vi "UPRcontroller_v00_basedonlsmv66.vi"() -> ()   [LabVIEW 2015] (continued)
                          tunnel: [_ _ _ _ _ w2450 _ _ _ _] -> w2290
                          tunnel: [_ _ _ _ _ w2449 _ _ _ _] -> w2289
                          tunnel: [_ _ _ _ _ w2448 _ _ _ _] -> w2288
                          tunnel: [_ _ _ _ _ w2447 _ _ _ _] -> w2287
                          tunnel: [_ _ _ _ _ w2446 _ _ _ _] -> w2286
                          tunnel: [_ _ _ _ _ w2445 _ _ _ _] -> w2285
                          tunnel: [_ _ _ _ _ w2444 _ _ _ _] -> w2284
                          tunnel: [_ _ _ _ _ w2443 _ _ _ _] -> w2283
                          frame #0 {
                            n108 = local read "Auto Shutter Channels"() -> (w2304:i32[])
                            n109 = local read "AI channels"() -> (w2310:i32[])
                            n110 = local read "CI channels"() -> (w2309:i32[])
                            n111 = call "2pparameters.vi"("command"="get") -> ("params out"=w2307:T12)  [unwired: 1 in]
                            n112 = Bundle By Name(cluster=w2307, "aAI"=w2310, "aCI"=w2309, "aAS"=w2304) -> (w2308:T12)
                            n113 = call "2pparameters.vi"("Params in"=w2308, "command"="set") -> ()  [unwired: 1 out]
                          }
                          frame #1 {
                            n114 = local read "Vy-min ref"() -> (w2315:dbl)
                            n115 = local read "Vy-max ref"() -> (w2316:dbl)
                            n116 = local read "Angle ref"() -> (w2314:dbl)
                            n117 = local read "Vx-min ref"() -> (w2317:dbl)
                            n118 = local write "counts"(0 ("counts")) -> ()
                            n119 = local write "graphtab"(T5."image" ("graphtab")) -> ()
                            n120 = local read "Vx-max ref"() -> (w2318:dbl)
                            n121 = property on="Stop" class="Bool (strict)"("Visible"=TRUE, "DisabledEnum"=T8."Enabled" ("Disabled")) -> ()  [unwired: 2 in, 2 out]
                            n122 = property on="Start" class="Bool (strict)"("Visible"=FALSE, "DisabledEnum"=T8."Disabled and Grayed Out" ("Disabled")) -> ()  [unwired: 2 in, 2 out]
                            n123 = script code="Xic=(ximax+ximin)./2;\nYic=(yimax+yimin)./2;\nximin=ximin-Xic;\nymin=ymin-Yic;\nxirmin=ximin.*cos(pi/180.*phi)+yimin.*sin(pi./180.*phi)+Xic;\nyirmin=-ximin.*sin(pi./180.*phi)+yimin.*cos(pi./180.*phi)+Yic;"("ximax"=w2318, "ximin"=w2317, "yimax"=w2316, "yimin"=w2315, "phi"=w2314) -> ("xirmin"=w2313:dbl, "yirmin"=w2312:dbl)  [unwired: 1 in, 1 out]
                            n124 = stacked-sequence {
                              tunnel: w2311 -> [_ w2343 _]
                              frame #0 {
                                n125 = local read "Measurement"() -> (w2325:T4)
                                n126 = case shown="\"X-Y-t movie\", Default" w2325 {
                                frame "X-Y-t movie", Default {
                                n127 = call "2pparameters.vi"("command"="get") -> ("params out"=w2328:T12)  [unwired: 1 in]
                                n128 = Bundle By Name(cluster=w2328, "type"="X-Y-t movie") -> (w2326:T12)
                                n129 = call "2pparameters.vi"("Params in"=w2326, "command"="set") -> ()  [unwired: 1 out]
                                }
                                frame "X-Y-Z stack" {
                                n130 = call "2pparameters.vi"("command"="get") -> ("params out"=w2333:T12)  [unwired: 1 in]
                                n131 = Bundle By Name(cluster=w2333, "type"="X-Y-Z stack") -> (w2331:T12)
                                n132 = call "2pparameters.vi"("Params in"=w2331, "command"="set") -> ()  [unwired: 1 out]
                                }
                                frame "Lifetime (scan)" {
                                n133 = call "2pparameters.vi"("command"="get") -> ("params out"=w2338:T12)  [unwired: 1 in]
                                n134 = Bundle By Name(cluster=w2338, "type"="Lifetime (scan)") -> (w2336:T12)
                                n135 = call "2pparameters.vi"("Params in"=w2336, "command"="set") -> ()  [unwired: 1 out]
                                }
                                }
                              }
                              frame #1 {
                                n136 = Format Date/Time String(time format string (%c)="%Y%m%d", seconds (now)=w2343) -> (date/time string=w2342:string)  [unwired: 1 in]
                                n137 = Format Date/Time String(time format string (%c)="%H%M%S", seconds (now)=w2343) -> (date/time string=w2341:string)  [unwired: 1 in]
                                n138 = call "2pparameters.vi"("command"="get") -> ("params out"=w2347:T12)  [unwired: 1 in]
                                n139 = Bundle By Name(cluster=w2347, "date"=w2342, "time"=w2341) -> (w2346:T12)
                                n140 = call "2pparameters.vi"("Params in"=w2346, "command"="set") -> ()  [unwired: 1 out]
                              }
                              frame #2 {
                                n141 = call "configuration.vi"("command"="get") -> ("config out"=w2357:T14)  [unwired: 2 in, 1 out]
                                n142 = Unbundle By Name(w2357) -> ("CI names"=w2358:string[], "AI names"=w2359:string[])
                                n143 = call "2pparameters.vi"("command"="get") -> ("params out"=w2353:T12)  [unwired: 1 in]
                                n144 = Unbundle By Name(w2353) -> ("aCI"=w2354:i32[], "aAI"=w2355:i32[])
                                n145 = for {
                                tunnel: w2354 -> [w2369] mode=indexing
                                tunnel: w2358 -> [w2370]
                                tunnel: [w2368] -> w2360 mode=indexing
                                n146 = Index Array(array=w2370, index=w2369) -> (element=w2368:string)
                                }
                                n147 = for {
                                tunnel: w2355 -> [w2366] mode=indexing
                                tunnel: w2359 -> [w2367]
                                tunnel: [w2365] -> w2361 mode=indexing
                                n148 = Index Array(array=w2367, index=w2366) -> (element=w2365:string)
                                }
                                n149 = Build Array (concatenate)(w2360, w2361) -> (w2351:string[])
                                n150 = for {
                                tunnel: w2351 -> [w2363] mode=indexing
                                tunnel: [w2362] -> w2350 mode=indexing
                                i -> [w2364]
                                n151 = Bundle("String"=w2363, w2364) -> (w2362:cluster{"String":string, i32})  [unwired: 1 in]
                                }
                                n152 = property on="image2list" class="Ring (strict)"("StringsAndValues[]"=w2350) -> ()  [unwired: 2 in, 2 out]
                                n153 = property on="image1list" class="Ring (strict)"("StringsAndValues[]"=w2350) -> ()  [unwired: 2 in, 2 out]
                                n154 = property on="image1list chB" class="Ring (strict)"("StringsAndValues[]"=w2350) -> ()  [unwired: 2 in, 2 out]
                                n155 = property on="image1list chA" class="Ring (strict)"("StringsAndValues[]"=w2350) -> ()  [unwired: 2 in, 2 out]
                              }
                            }
                            n156 = call "setposition.vi"("Vy"=w2312, "Vx"=w2313) -> ()  [unwired: 1 in]
                          }
                          frame #2 {
                            n157 = call "X-array-databuffer.vi"("command"=enum16{"get", "set", "clear", "append"}."clear") -> ()  [unwired: 3 in, 2 out]
                            n158 = call "Y-array-databuffer.vi"("command"=enum16{"get", "set", "clear", "append"}."clear") -> ()  [unwired: 3 in, 2 out]
                            n159 = call "2pparameters.vi"("command"="get") -> ("params out"=w2374:T12)  [unwired: 1 in]
                            n160 = Unbundle By Name(w2374) -> ("aAS"=w2371:u32[], "autoshutter"=w2375:bool, "auto OD"=w2372:bool)
                            n161 = call "allAI-temp_img.vi"("command"=enum16{"get", "set", "clear", "append"}."clear") -> ()  [unwired: 3 in, 2 out]
                            n162 = case shown="True" w2372 {
                              frame False {
                              }
                              frame True {
                                n163 = call "configuration.vi"("command"="get") -> ("config out"=w2383:T14)  [unwired: 2 in, 1 out]
                                n164 = Unbundle By Name(w2383) -> ("image OD"=w2384:u16)
                                n165 = local read "ODfilt"() -> (w2381:u16)
                                n166 = call "filterwheelcontrol_nothorlabslib.vi"("Current OD filt"=w2381, "New ODfilt"=w2384) -> ()  [unwired: 1 in]
                              }
                            }
                            n167 = case shown="True" w2375 {
                              tunnel: w2371 -> [_ w2385]
                              frame False {
                              }
                              frame True {
                                n168 = call "shuttercontrol_multi.vi"("Autoshutter Chans"=w2385, "command"="close") -> ()  [unwired: 1 in, 1 out]
                              }
                            }
                            n169 = call "CH1-temp.vi"("command"=enum16{"get", "set", "clear", "add row"}."clear") -> ()  [unwired: 3 in, 2 out]
                            n170 = call "CH2-temp.vi"("command"=enum16{"get", "set", "clear", "add row"}."clear") -> ()  [unwired: 3 in, 2 out]
                          }
                          frame #3 {
                            n171 = local read "avpp"() -> (w2419:i32)
                            n172 = local read "Angle ref"() -> (w2418:dbl)
                            n173 = local read "ROI Type"() -> (w2417:u16)
                            n174 = local read "xpixels ref"() -> (w2414:i32)
                            n175 = local read "Vx-min ref"() -> (w2413:dbl)
                            n176 = local read "Vx-max ref"() -> (w2412:dbl)
                            n177 = local read "ypixels ref"() -> (w2410:i32)
                            n178 = local read "Vy-min ref"() -> (w2411:dbl)
                            n179 = local read "Vy-max ref"() -> (w2407:dbl)
                            n180 = local read "Sampling rate"() -> (w2401:dbl)
                            n181 = local read "finite samples"() -> (w2402:bool)
                            n182 = local read "continuous"() -> (w2405:bool)
                            n183 = local read "wavdet"() -> (w2406:bool)
                            n184 = local read "# of frames"() -> (w2404:i32)
                            n185 = local read "maxbufferAI"() -> (w2403:i32)
                            n186 = local read "Override AI buffer"() -> (w2387:bool)
                            n187 = call "2pparameters.vi"("command"="get") -> ("params out"=w2416:T12)  [unwired: 1 in]
                            n188 = Bundle By Name(cluster=w2416, "avpp"=w2419, "Angle Img"=w2418, "Xpixels Img"=w2414, "Vx-min Img"=w2413, "VX-max Img"=w2412, "Ypixels Img"=w2410, "Vy-min Img"=w2411, "Vy-max Img"=w2407, "srate"=w2401, "srate Img"=w2401, "finite"=w2402, "cont"=w2405, "wavdet"=w2406, "measpoints"=w2404, "maxbufferAI"=w2403, "Drawing Mode"=w2417, "Vz-reset"=0.0, "AIoverride"=w2387) -> (w2408:T12)
                            n189 = call "2pparameters.vi"("Params in"=w2408, "command"="set") -> ()  [unwired: 1 out]
                            n190 = local read "Vholding (mV)"() -> (w2390:sgl)
                            n191 = local read "OCgain"() -> (w2391:sgl)
                            n192 = local read "holdon"() -> (w2389:bool)
                            n193 = local read "Current Clamp"() -> (w2396:bool)
                            n194 = local read "Voltage Clamp"() -> (w2395:bool)
                            n195 = local read "CC_ICgain"() -> (w2394:dbl)
                            n196 = call "patchparameters.vi"("command"="get") -> ("Params out"=w2398:T16)  [unwired: 1 in]
                            n197 = Bundle By Name(cluster=w2398, "VC"=w2395, "CC"=w2396, "CC_icg (pA/mv)"=w2394, "VC_icg (mV/mV)"=sgl 10.0, "OCG (mV/pA)"=w2391, "OVG (mV/mV)"=0.1, "Vhold (mV)"=w2390, "holdon"=w2389) -> (w2397:T16)
                            n198 = call "patchparameters.vi"("Params in"=w2397, "command"="set") -> ()  [unwired: 1 out]
                          }
                          frame #4 {
                            # "these store the actual scanning waveforms (for one iteration)"
                            # "Generate Waveforms for Scanning Mirrors"
                            # "Creates The scanning waveform here"
                            n199 = call "2pparameters.vi"("command"="get") -> ("params out"=w2434:T12)  [unwired: 1 in]
                            n200 = Unbundle By Name(w2434) -> ("srate Img"=w2433:sgl, "Angle Img"=w2432:dbl, "VX-max Img"=w2431:dbl, "Vx-min Img"=w2430:dbl, "Xpixels Img"=w2429:i32, "Ypixels Img"=w2428:i32, "Vy-max Img"=w2427:dbl, "Vy-min Img"=w2426:dbl, "Drawing Mode"=w2425:u16)
                            n201 = call "ROI-databuffer.vi"("command"=enum16{"get", "set", "clear", "append"}."get") -> ("array out"=w2424:cluster{"x":sgl, "y":sgl}[])  [unwired: 4 in]
                            n202 = call "ScanningWaveform_v4.vi"("Vy-min"=w2426, "Vy-max"=w2427, "yPixels/tPixels"=w2428, "xPixels/rPixels"=w2429, "Vx-min"=w2430, "Vx-max"=w2431, "Drawing Mode"=w2425, "Angle"=w2432, "AOrate"=w2433, "Points"=w2424) -> ("numPixels"=w2420:dbl, "Y-WaveArray"=w2423:dbl[], "P"=w2421:dbl, "X-WaveArray"=w2422:dbl[])  [unwired: 6 in]
                            n203 = call "2pparameters.vi"("command"="get") -> ("params out"=w2442:T12)  [unwired: 1 in]
                            n204 = call "Y-array-databuffer.vi"("array in"=w2423, "command"=enum16{"get", "set", "clear", "append"}."set") -> ()  [unwired: 2 in, 2 out]
                            n205 = call "X-array-databuffer.vi"("array in"=w2422, "command"=enum16{"get", "set", "clear", "append"}."set") -> ()  [unwired: 2 in, 2 out]
                            n206 = Bundle By Name(cluster=w2442, "P"=w2421, "sAOxy"=w2420) -> (w2439:T12)
                            n207 = call "2pparameters.vi"("Params in"=w2439, "command"="set") -> ()  [unwired: 1 out]
                          }
                          frame #5 {
                            # "rem2Ps"
                            # "A2Ps"
                            # "Al"
                            # "Rl"
                            # "Combines scanning waveform with \"wavform generation\" waveforms"
                            n208 = stacked-sequence {
                              seq-local: [w2461 _ _ _ _ _ _ _ _ _ _] -> [_ w2581 _ w2636 _ w2716 _ _ _ _ _]
                              seq-local: [w2462 _ _ _ _ _ _ _ _ _ _] -> [_ w2582 w2592 _ w2685 _ _ _ _ _ _]
                              seq-local: [_ _ w2591 _ _ _ _ _ _ _ _] -> [_ _ _ _ w2679 _ _ _ _ _ _]
                              seq-local: [_ _ _ w2635 _ _ _ _ _ _ _] -> [_ _ _ _ _ w2715 _ _ _ _ _]
                              seq-local: [w2458 _ _ _ _ _ _ _ _ _ _] -> [_ w2578 _ _ _ _ _ _ w2925 w2993 _]
                              seq-local: [w2457 _ _ _ _ _ _ _ _ _ _] -> [_ w2577 _ _ _ _ _ _ w2926 w2994 _]
                              seq-local: [w2464 _ _ _ _ _ _ _ _ _ _] -> [_ _ _ _ _ _ w2754 _ w2924 w2992 _]
                              seq-local: [w2460 _ _ _ _ _ _ _ _ _ _] -> [_ w2576 _ _ _ _ w2753 w2832 _ _ _]
                              seq-local: [w2459 _ _ _ _ _ _ _ _ _ _] -> [_ w2575 _ _ _ _ w2752 w2831 _ _ _]
                              seq-local: [w2463 _ _ _ _ _ _ _ _ _ _] -> [_ _ _ _ _ _ w2751 w2830 _ _ _]
                              tunnel: [_ _ w2590 _ _ _ _ _ _ _ _] -> w2455
                              tunnel: [_ _ w2589 _ _ _ _ _ _ _ _] -> w2454
                              tunnel: [w2462 _ _ _ _ _ _ _ _ _ _] -> w2456
                              tunnel: [w2461 _ _ _ _ _ _ _ _ _ _] -> w2453
                              tunnel: [_ _ _ w2634 _ _ _ _ _ _ _] -> w2452
                              tunnel: [_ _ _ w2633 _ _ _ _ _ _ _] -> w2451
                              tunnel: [w2460 _ _ _ _ _ _ _ _ _ _] -> w2450
                              tunnel: [w2459 _ _ _ _ _ _ _ _ _ _] -> w2449
                              tunnel: [_ _ _ _ _ _ w2750 _ _ _ _] -> w2448
                              tunnel: [_ _ _ _ _ _ _ w2829 _ _ _] -> w2447
                              tunnel: [w2458 _ _ _ _ _ _ _ _ _ _] -> w2446
                              tunnel: [w2457 _ _ _ _ _ _ _ _ _ _] -> w2445
                              tunnel: [_ _ _ _ _ _ _ _ w2923 _ _] -> w2444
                              tunnel: [_ _ _ _ _ _ _ _ _ w2991 _] -> w2443
                              frame #0 {
                                # "channels\nadded/removed"
                                # "all these arrows go to frames\n6 and 7"
                                # "for a next version, give ome thought to\nthe possibilit of intermittently updating the\nwaveforms. it will have to be a calculation\nbased on speed of CPU and program on the one hand\nand length of measurement on the other. but then it should be possible, in principle, to \nupdate the waveform on the fly and that way cut up a longer measurement in smaller parts."
                                # "Y"
                                # "X"
                                # "This frame takes channels from \"waveform generation\" and adds, X,Y,2p shutter and Lifetime Timestamp (if those where not manually defined in WG)"
                                n209 = stacked-sequence {
                                tunnel: [w2465 _ _ _] -> w2462
                                tunnel: [_ w2477 _ _] -> w2461
                                tunnel: [_ _ _ w2542] -> w2457
                                tunnel: [_ _ _ w2541] -> w2458
                                tunnel: [_ _ _ w2540] -> w2464
                                tunnel: [_ _ w2492 _] -> w2460
                                tunnel: [_ _ w2491 _] -> w2459
                                tunnel: [_ _ w2490 _] -> w2463
                                frame #0 {
                                n210 = call "configuration.vi"("command"="get") -> ("config out"=w2467:T14)  [unwired: 2 in, 1 out]
                                n211 = Unbundle By Name(w2467) -> ("Voltage to Xgalvo"=w2466:i32)
                                n212 = call "2pparameters.vi"("command"="get") -> ("params out"=w2471:T12)  [unwired: 1 in]
                                n213 = in-place {
                                in-place-border: w2466 -> [w2476]
                                in-place-border: [w2473] -> w2465
                                n214 = in-place-cluster #1(w2471) -> ("aAO"=w2475:u32[])
                                n215 = call "add channel to active arrayv2.vi"("line array in"=w2475, "line to add"=w2476) -> ("line array out"=w2474:u32[], "addition"=w2473:bool)  [unwired: 1 out]
                                n216 = in-place-cluster #1("aAO"=w2474) -> (w2469:T12)
                                }
                                n217 = call "2pparameters.vi"("Params in"=w2469, "command"="set") -> ()  [unwired: 1 out]
                                }
                                frame #1 {
                                n218 = call "configuration.vi"("command"="get") -> ("config out"=w2479:T14)  [unwired: 2 in, 1 out]
                                n219 = Unbundle By Name(w2479) -> ("Voltage to Ygalvo"=w2478:i32)
                                n220 = call "2pparameters.vi"("command"="get") -> ("params out"=w2483:T12)  [unwired: 1 in]
                                n221 = in-place {
                                in-place-border: w2478 -> [w2488]
                                in-place-border: [w2485] -> w2477
                                n222 = in-place-cluster #2(w2483) -> ("aAO"=w2487:u32[])
                                n223 = call "add channel to active arrayv2.vi"("line array in"=w2487, "line to add"=w2488) -> ("line array out"=w2486:u32[], "addition"=w2485:bool)  [unwired: 1 out]
                                n224 = in-place-cluster #2("aAO"=w2486) -> (w2481:T12)
                                }
                                n225 = call "2pparameters.vi"("Params in"=w2481, "command"="set") -> ()  [unwired: 1 out]
                                }
                                frame #2 {
                                n226 = call "2pparameters.vi"("command"="get") -> ("params out"=w2494:T12)  [unwired: 1 in]
                                n227 = Unbundle By Name(w2494) -> ("autoshutter"=w2493:bool, "wavdet"=w2489:bool)
                                n228 = case shown="False" w2493 {
                                tunnel: [w2499 w2522] -> w2492
                                tunnel: [w2498 FALSE ("removal")] -> w2491
                                tunnel: [w2497 w2521] -> w2490
                                tunnel: w2489 -> [w2496 _]
                                frame False {
                                n229 = case shown="False" w2496 {
                                tunnel: [FALSE ("addition") FALSE ("addition")] -> w2499
                                tunnel: [w2503 FALSE ("removal")] -> w2498
                                tunnel: [w2502 _] -> w2497
                                frame False {
                                n230 = call "2pparameters.vi"("command"="get") -> ("params out"=w2501:T12)  [unwired: 1 in]
                                n231 = Unbundle By Name(w2501) -> ("aAS"=w2500:u32[])
                                n232 = in-place {
                                in-place-border: [w2508] -> w2503
                                in-place-border: [w2511] -> w2502
                                in-place-border: w2500 -> [w2510]
                                n233 = in-place-cluster #3(w2501) -> ("aDO"=w2513:u32[])
                                n234 = for {
                                tunnel: [w2516] -> w2509 mode=indexing
                                tunnel: [w2515] -> w2511 mode=indexing
                                shift-right: [w2517] -> w2512
                                shift-left: w2513 -> [w2518]
                                tunnel: w2510 -> [w2514] mode=indexing
                                n235 = call "remove channel from active arrayv2.vi"("line array in"=w2518, "line to remove"=w2514) -> ("line array out"=w2517:u32[], "removal"=w2516:bool, "index"=w2515:i32)
                                }
                                n236 = Or Array Elements(Boolean array=w2509) -> (logical OR=w2508:bool)
                                n237 = in-place-cluster #3("aDO"=w2512) -> (w2504:T12)
                                }
                                n238 = call "2pparameters.vi"("Params in"=w2504, "command"="set") -> ()  [unwired: 1 out]
                                }
                                frame True {
                                }
                                }
                                }
                                frame True {
                                n239 = call "2pparameters.vi"("command"="get") -> ("params out"=w2524:T12)  [unwired: 1 in]
                                n240 = Unbundle By Name(w2524) -> ("aAS"=w2523:u32[])
                                n241 = in-place {
                                in-place-border: w2523 -> [w2534]
                                in-place-border: [w2530] -> w2522
                                in-place-border: [w2529] -> w2521
                                n242 = in-place-cluster #4(w2524) -> ("aDO"=w2533:u32[])
                                n243 = for {
                                tunnel: w2534 -> [w2539] mode=indexing
                                shift-right: [w2537] -> w2532
                                shift-left: w2533 -> [w2538]
                                tunnel: [w2536] -> w2531 mode=indexing
                                tunnel: [w2535] -> w2529 mode=indexing
                                n244 = call "add channel to active arrayv2.vi"("line array in"=w2538, "line to add"=w2539) -> ("line array out"=w2537:u32[], "addition"=w2536:bool, "index"=w2535:i32)
                                }
                                n245 = Or Array Elements(Boolean array=w2531) -> (logical OR=w2530:bool)
                                n246 = in-place-cluster #4("aDO"=w2532) -> (w2526:T12)
                                }
                                n247 = call "2pparameters.vi"("Params in"=w2526, "command"="set") -> ()  [unwired: 1 out]
                                }
                                }
                                }
                                frame #3 {
                                n248 = local read "Measurement"() -> (w2543:T4)
                                n249 = To Unsigned Long Integer(number=w2543) -> (unsigned 32bit integer=w2544:u32)
                                n250 = case shown="5..7" w2544 {
                                tunnel: [FALSE ("addition") w2562] -> w2542
                                tunnel: [w2547 FALSE ("removal")] -> w2541
                                tunnel: [w2545 w2560] -> w2540
                                frame 0..4, Default {
                                n251 = call "configuration.vi"("command"="get") -> ("config out"=w2553:T14)  [unwired: 2 in, 1 out]
                                n252 = Unbundle By Name(w2553) -> ("LT timestamp"=w2550:u32)
                                n253 = call "2pparameters.vi"("command"="get") -> ("params out"=w2551:T12)  [unwired: 1 in]
                                n254 = in-place {
                                in-place-border: w2550 -> [w2559]
                                in-place-border: [w2556] -> w2547
                                in-place-border: [w2555] -> w2545
                                n255 = in-place-cluster #5(w2551) -> ("aDO"=w2558:u32[])
                                n256 = call "remove channel from active arrayv2.vi"("line array in"=w2558, "line to remove"=w2559) -> ("line array out"=w2557:u32[], "removal"=w2556:bool, "index"=w2555:i32)
                                n257 = in-place-cluster #5("aDO"=w2557) -> (w2548:T12)
                                }
                                n258 = call "2pparameters.vi"("Params in"=w2548, "command"="set") -> ()  [unwired: 1 out]
                                }
                                frame 5..7 {
                                n259 = call "configuration.vi"("command"="get") -> ("config out"=w2568:T14)  [unwired: 2 in, 1 out]
                                n260 = Unbundle By Name(w2568) -> ("LT timestamp"=w2565:u32)
                                n261 = call "2pparameters.vi"("command"="get") -> ("params out"=w2566:T12)  [unwired: 1 in]
                                n262 = in-place {
                                in-place-border: w2565 -> [w2574]
                                in-place-border: [w2571] -> w2562
                                in-place-border: [w2570] -> w2560
                                n263 = in-place-cluster #6(w2566) -> ("aDO"=w2573:u32[])
                                n264 = call "add channel to active arrayv2.vi"("line array in"=w2573, "line to add"=w2574) -> ("line array out"=w2572:u32[], "addition"=w2571:bool, "index"=w2570:i32)
                                n265 = in-place-cluster #6("aDO"=w2572) -> (w2563:T12)
                                }
                                n266 = call "2pparameters.vi"("Params in"=w2563, "command"="set") -> ()  [unwired: 1 out]
                                }
                                }
                                }
                                }
                              }
                              frame #1 {
                                # "Prepares the actual AO and DO lines that are going to be used for the task"
                                n267 = Or(x=w2581, y=w2582) -> (x .or. y?=w2580:bool)
                                n268 = case shown="True" w2580 {
                                frame False {
                                }
                                frame True {
                                # "update GUI"
                                n269 = call "Used AO lines.vi"() -> ("used AO names"=w2586:string[], "used AO lines"=w2588:tag[])  [unwired: 2 in]
                                n270 = control-ref of="Analog Lines Plot"() -> (w2587:refnum<vi>)
                                n271 = local write "Analog Used Lines"(w2588) -> ()
                                n272 = local write "Analog Used Names"(w2586) -> ()
                                n273 = call "prepAOWaveplot.vi"("WaveformGraph in"=w2587, "Analog Used Names"=w2586) -> ()  [unwired: 1 in]
                                }
                                }
                                n274 = Compound Arithmetic op=OR(w2578, w2577, w2576, w2575) -> (w2579:bool)
                                n275 = case shown="True" w2579 {
                                frame False {
                                }
                                frame True {
                                n276 = control-ref of="Digital Lines Plot"() -> (w2583:refnum<vi>)
                                n277 = call "Used DO lines.vi"() -> ("used DO names"=w2584:string[], "used DO lines"=w2585:tag[])  [unwired: 2 in]
                                n278 = local write "Digital Used Lines"(w2585) -> ()
                                n279 = local write "Digital Used Names"(w2584) -> ()
                                n280 = call "prepDOWaveplot.vi"("DigitalGraph in"=w2583, "used DO names"=w2584) -> ()  [unwired: 1 in]
                                }
                                }
                              }
                              frame #2 {
                                # "Make sure that the parameters used to create waveform are saved in the right format"
                                n281 = case shown="False" w2592 {
                                tunnel: [w2595 w2616] -> w2591
                                tunnel: [w2594 w2614] -> w2590
                                tunnel: [w2593 _] -> w2589
                                frame False {
                                n282 = stacked-sequence {
                                seq-local: [w2597 _] -> [_ w2610]
                                tunnel: [w2597 _] -> w2595
                                tunnel: [w2600 _] -> w2594
                                tunnel: [w2596 _] -> w2593
                                frame #0 {
                                n283 = call "configuration.vi"("command"="get") -> ("config out"=w2608:T14)  [unwired: 2 in, 1 out]
                                n284 = call "waveformparamsv2.vi"("command"="get") -> ("Params out"=w2602:T17)  [unwired: 4 in, 2 out]
                                n285 = Unbundle By Name(w2608) -> ("Voltage to Xgalvo"=w2609:i32)
                                n286 = call "2pparameters.vi"("command"="get") -> ("params out"=w2605:T12)  [unwired: 1 in]
                                n287 = Unbundle By Name(w2602) -> ("AO parameters"=w2601:T18)
                                n288 = Unbundle By Name(w2605) -> ("aAO"=w2606:u32[])
                                n289 = call "waveformsAObuffer.vi"("command"="get") -> ("AO wf out"=w2598:waveform(dbl)[])  [unwired: 1 in]
                                n290 = Search 1D Array(1D array=w2606, element=w2609) -> (index of element=w2597:i32)  [unwired: 1 in]
                                n291 = Index Array(array=w2598, index=w2597) -> (element=w2596:waveform(dbl))
                                n292 = Index Array(array=w2601, index=w2597) -> (element=w2600:T19)
                                }
                                frame #1 {
                                w2611 = 0.0 ("Step size (V)")
                                n293 = local read "Sampling rate"() -> (w2612:dbl)
                                n294 = call "replace AO XYwfparam.vi"("Baseline (V)"=w2611, "Start amplitude (V)"=w2611, "Cycles"=w2611, "Repeats"=w2611, "index of AO wave"=w2610, "Step size (V)"=w2611, "DC (%)"=w2611, "Sampling frequency (Hz)"=w2612, "Period (ms)"=w2611, "Cycle length (s)"=w2611, "Pulses"=w2611, "padding value"=w2611, "Matlab wave name"=path "xwave") -> ()  [unwired: 3 in]
                                }
                                }
                                }
                                frame True {
                                w2615 = 0.0 ("Repeats")
                                n295 = local read "Sampling rate"() -> (w2624:dbl)
                                n296 = call "2pparameters.vi"("command"="get") -> ("params out"=w2618:T12)  [unwired: 1 in]
                                n297 = call "configuration.vi"("command"="get") -> ("config out"=w2621:T14)  [unwired: 2 in, 1 out]
                                n298 = call "waveformparamsv2.vi"("command"="get") -> ("Params out"=w2630:T17)  [unwired: 4 in, 2 out]
                                n299 = Unbundle By Name(w2621) -> ("Voltage to Xgalvo"=w2622:i32)
                                n300 = Unbundle By Name(w2630) -> ("AO parameters"=w2627:T18)
                                n301 = Unbundle By Name(w2618) -> ("aAO"=w2619:u32[])
                                n302 = Search 1D Array(1D array=w2619, element=w2622) -> (index of element=w2616:i32)  [unwired: 1 in]
                                n303 = Index Array(array=w2627, index=0) -> (element=w2628:T19)
                                n304 = Bundle By Name(cluster=w2628, "AOtab"=-1.0 ("Repeats"), "Repeats"=w2615, "Cycles"=w2615, "Start amplitude (V)"=w2615, "Baseline (V)"=w2615, "Step size (V)"=w2615, "DC (%)"=w2615, "Sampling frequency (Hz)"=w2624, "Period (ms)"=w2615, "Offset (V)"=w2615, "Amplitude (V)"=w2615, "Frequency"=w2615, "Tri Repeats"=w2615, "phase shift (ms)"=w2615, "Pulses"=w2615, "Matlab wave file"=path "xwave", "padding value"=w2615) -> (w2614:T19)
                                n305 = Build Array(w2614) -> (w2625:T18)
                                n306 = call "waveformparamsv2.vi"("command"="add AO", "add AO"=w2625) -> ()  [unwired: 3 in, 3 out]
                                }
                                }
                              }
                              frame #3 {
                                n307 = case shown="False" w2636 {
                                tunnel: [w2639 w2660] -> w2635
                                tunnel: [w2638 w2658] -> w2634
                                tunnel: [w2637 _] -> w2633
                                frame False {
                                n308 = stacked-sequence {
                                seq-local: [w2641 _] -> [_ w2654]
                                tunnel: [w2641 _] -> w2639
                                tunnel: [w2644 _] -> w2638
                                tunnel: [w2640 _] -> w2637
                                frame #0 {
                                n309 = call "configuration.vi"("command"="get") -> ("config out"=w2652:T14)  [unwired: 2 in, 1 out]
                                n310 = call "waveformparamsv2.vi"("command"="get") -> ("Params out"=w2646:T17)  [unwired: 4 in, 2 out]
                                n311 = Unbundle By Name(w2652) -> ("Voltage to Ygalvo"=w2653:i32)
                                n312 = call "2pparameters.vi"("command"="get") -> ("params out"=w2649:T12)  [unwired: 1 in]
                                n313 = Unbundle By Name(w2646) -> ("AO parameters"=w2645:T18)
                                n314 = Unbundle By Name(w2649) -> ("aAO"=w2650:u32[])
                                n315 = call "waveformsAObuffer.vi"("command"="get") -> ("AO wf out"=w2642:waveform(dbl)[])  [unwired: 1 in]
                                n316 = Search 1D Array(1D array=w2650, element=w2653) -> (index of element=w2641:i32)  [unwired: 1 in]
                                n317 = Index Array(array=w2642, index=w2641) -> (element=w2640:waveform(dbl))
                                n318 = Index Array(array=w2645, index=w2641) -> (element=w2644:T19)
                                }
                                frame #1 {
                                w2655 = 0.0 ("Step size (V)")
                                n319 = local read "Sampling rate"() -> (w2656:dbl)
                                n320 = call "replace AO XYwfparam.vi"("Baseline (V)"=w2655, "Start amplitude (V)"=w2655, "Cycles"=w2655, "Repeats"=w2655, "index of AO wave"=w2654, "Step size (V)"=w2655, "DC (%)"=w2655, "Sampling frequency (Hz)"=w2656, "Period (ms)"=w2655, "Cycle length (s)"=w2655, "Pulses"=w2655, "padding value"=w2655, "Matlab wave name"=path "ywave") -> ()  [unwired: 3 in]
                                }
                                }
                                }
                                frame True {
                                w2659 = 0.0 ("Repeats")
                                n321 = local read "Sampling rate"() -> (w2669:dbl)
                                n322 = call "2pparameters.vi"("command"="get") -> ("params out"=w2662:T12)  [unwired: 1 in]
                                n323 = call "configuration.vi"("command"="get") -> ("config out"=w2665:T14)  [unwired: 2 in, 1 out]
                                n324 = call "waveformparamsv2.vi"("command"="get") -> ("Params out"=w2675:T17)  [unwired: 4 in, 2 out]
                                n325 = Unbundle By Name(w2665) -> ("Voltage to Ygalvo"=w2666:i32)
                                n326 = Unbundle By Name(w2675) -> ("AO parameters"=w2672:T18)
                                n327 = Unbundle By Name(w2662) -> ("aAO"=w2663:u32[])
                                n328 = Search 1D Array(1D array=w2663, element=w2666) -> (index of element=w2660:i32)  [unwired: 1 in]
                                n329 = Index Array(array=w2672, index=0) -> (element=w2673:T19)
                                n330 = Bundle By Name(cluster=w2673, "AOtab"=-1.0 ("Repeats"), "Repeats"=w2659, "Cycles"=w2659, "Start amplitude (V)"=w2659, "Baseline (V)"=w2659, "Step size (V)"=w2659, "DC (%)"=w2659, "Sampling frequency (Hz)"=w2669, "Period (ms)"=w2659, "Offset (V)"=w2659, "Amplitude (V)"=w2659, "Frequency"=w2659, "Tri Repeats"=w2659, "phase shift (ms)"=w2659, "Pulses"=w2659, "Matlab wave file"=path "ywave", "padding value"=w2659) -> (w2658:T19)
                                n331 = Build Array(w2658) -> (w2670:T18)
                                n332 = call "waveformparamsv2.vi"("command"="add AO", "add AO"=w2670) -> ()  [unwired: 3 in, 3 out]
                                }
                                }
                              }
                              frame #4 {
                                # "Create waveforms for X"
                                n333 = call "2pparameters.vi"("command"="get") -> ("params out"=w2682:T12)  [unwired: 1 in]
                                n334 = Unbundle By Name(w2682) -> ("wavdet"=w2681:bool, "sAOxy"=w2678:i32, "refwfsize"=w2677:dbl, "srate Img"=w2680:sgl)
                                n335 = case shown="True" w2681 {
                                tunnel: [w2686 w2696] -> w2684
                                tunnel: w2680 -> [w2687 w2698]
                                tunnel: w2678 -> [_ w2694]
                                tunnel: w2677 -> [_ w2693]
                                frame False {
                                n336 = call "X-array-databuffer.vi"("command"=enum16{"get", "set", "clear", "append"}."get") -> ("array out"=w2690:dbl[])  [unwired: 3 in, 1 out]
                                n337 = Reciprocal(x=w2687) -> (1/x=w2688:sgl)
                                n338 = Bundle By Name("Y"=w2690, "dt"=w2688) -> (w2686:waveform(dbl))  [unwired: 1 in]
                                }
                                frame True {
                                n339 = To Double Precision Float(number=w2694) -> (double precision float=w2695:dbl)
                                n340 = Divide(x=w2693, y=w2695) -> (x/y=w2691:dbl)
                                n341 = Round Toward +Infinity(x=w2691) -> (ceil(x): smallest int >= x=w2692:dbl)
                                n342 = call "X-array-databuffer.vi"("command"=enum16{"get", "set", "clear", "append"}."get") -> ("array out"=w2700:dbl[])  [unwired: 3 in, 1 out]
                                n343 = Reciprocal(x=w2698) -> (1/x=w2699:sgl)
                                n344 = for {
                                N: w2692 -> [_]
                                tunnel: w2700 -> [w2702]
                                tunnel: [w2702] -> w2697 mode=concatenating
                                }
                                n345 = Bundle By Name("Y"=w2697, "dt"=w2699) -> (w2696:waveform(dbl))  [unwired: 1 in]
                                }
                                }
                                n346 = case shown="True" w2685 {
                                tunnel: w2684 -> [w2704 w2710]
                                tunnel: w2679 -> [w2705 _]
                                frame False {
                                n347 = call "waveformsAObuffer.vi"("command"="get") -> ("AO wf out"=w2708:waveform(dbl)[])  [unwired: 1 in]
                                n348 = Replace Array Subset(array=w2708, new element=w2704, index=w2705) -> (w2703:waveform(dbl)[])
                                n349 = call "waveformsAObuffer.vi"("AO wf in"=w2703, "command"="set") -> ()  [unwired: 1 out]
                                }
                                frame True {
                                n350 = call "waveformsAObuffer.vi"("command"="get") -> ("AO wf out"=w2712:waveform(dbl)[])  [unwired: 1 in]
                                n351 = Build Array (concatenate)(w2712, w2710) -> (w2709:waveform(dbl)[])
                                n352 = call "waveformsAObuffer.vi"("AO wf in"=w2709, "command"="set") -> ()  [unwired: 1 out]
                                }
                                }
                              }
                              frame #5 {
                                # "... and create waveform for Y"
                                n353 = call "2pparameters.vi"("command"="get") -> ("params out"=w2724:T12)  [unwired: 1 in]
                                n354 = Unbundle By Name(w2724) -> ("wavdet"=w2723:bool, "sAOxy"=w2721:i32, "refwfsize"=w2722:dbl, "srate Img"=w2717:sgl)
                                n355 = To Double Precision Float(number=w2721) -> (double precision float=w2720:dbl)
                                n356 = Divide(x=w2722, y=w2720) -> (x/y=w2719:dbl)
                                n357 = Round Toward +Infinity(x=w2719) -> (ceil(x): smallest int >= x=w2718:dbl)
                                n358 = case shown="False" w2723 {
                                tunnel: [w2728 w2733] -> w2714
                                tunnel: w2718 -> [_ w2737]
                                tunnel: w2717 -> [w2729 w2735]
                                frame False {
                                n359 = call "Y-array-databuffer.vi"("command"=enum16{"get", "set", "clear", "append"}."get") -> ("array out"=w2726:dbl[])  [unwired: 3 in, 1 out]
                                n360 = Reciprocal(x=w2729) -> (1/x=w2730:sgl)
                                n361 = Bundle By Name("Y"=w2726, "dt"=w2730) -> (w2728:waveform(dbl))  [unwired: 1 in]
                                }
                                frame True {
                                # "Tile the waveform N times if wavefrom generation is being used"
                                n362 = call "Y-array-databuffer.vi"("command"=enum16{"get", "set", "clear", "append"}."get") -> ("array out"=w2731:dbl[])  [unwired: 3 in, 1 out]
                                n363 = Reciprocal(x=w2735) -> (1/x=w2736:sgl)
                                n364 = for {
                                N: w2737 -> [_]
                                tunnel: w2731 -> [w2738]
                                tunnel: [w2738] -> w2734 mode=concatenating
                                }
                                n365 = Bundle By Name("Y"=w2734, "dt"=w2736) -> (w2733:waveform(dbl))  [unwired: 1 in]
                                }
                                }
                                n366 = case shown="False" w2716 {
                                tunnel: w2714 -> [w2741 w2746]
                                tunnel: w2715 -> [w2742 _]
                                frame False {
                                # "Add (tiled) waveform to the full set of waveforms forAO"
                                n367 = call "waveformsAObuffer.vi"("command"="get") -> ("AO wf out"=w2744:waveform(dbl)[])  [unwired: 1 in]
                                n368 = Replace Array Subset(array=w2744, new element=w2741, index=w2742) -> (w2739:waveform(dbl)[])
                                n369 = call "waveformsAObuffer.vi"("AO wf in"=w2739, "command"="set") -> ()  [unwired: 1 out]
                                }
                                frame True {
                                n370 = call "waveformsAObuffer.vi"("command"="get") -> ("AO wf out"=w2748:waveform(dbl)[])  [unwired: 1 in]
                                n371 = Build Array (concatenate)(w2748, w2746) -> (w2745:waveform(dbl)[])
                                n372 = call "waveformsAObuffer.vi"("AO wf in"=w2745, "command"="set") -> ()  [unwired: 1 out]
                                }
                                }
                              }
                              frame #6 {
                                # "Calculate  waveform for the 2p shutter to the digital waveforms (4 possibilities of whether it is there and if it needs to be there)"
                                n373 = Build Array(w2753, w2752) -> (w2756:bool[])
                                n374 = Boolean Array To Number(Boolean array=w2756) -> (number=w2755:u32)
                                n375 = case shown="0" w2755 {
                                tunnel: w2754 -> [_ _ _ _]
                                tunnel: w2751 -> [w2760 w2781 _ w2799]
                                tunnel: [_ w2780 _ w2797] -> w2750
                                frame 1 {
                                w2770 = 0.0 ("DOtab")
                                # "remove True; add False"
                                n376 = call "2pparameters.vi"("command"="get") -> ("params out"=w2767:T12)  [unwired: 1 in]
                                n377 = call "waveformparamsv2.vi"("command"="get") -> ("Params out"=w2776:T17)  [unwired: 4 in, 2 out]
                                n378 = Unbundle By Name(w2776) -> ("DO parameters"=w2774:T20)
                                n379 = Unbundle By Name(w2767) -> ("srate"=w2763:sgl, "sAOxy"=w2766:i32)
                                n380 = To Double Precision Float(number=w2763) -> (double precision float=w2761:dbl)
                                n381 = To Double Precision Float(number=w2763) -> (double precision float=w2762:dbl)
                                n382 = To Double Precision Float(number=w2766) -> (double precision float=w2765:dbl)
                                n383 = Divide(x=w2762, y=w2765) -> (x/y=w2764:dbl)
                                n384 = Index Array(array=w2774, index=0) -> (element=w2773:T21)
                                n385 = Bundle By Name(cluster=w2773, "Digital DC (%)"=100.0, "Digital phase"=w2770, "Digital Freq (Hz)"=w2764, "Sampling frequency (Hz)"=w2761, "Digital time offset (s)"=w2770, "padding value"=0.0, "matlab wave file"=path "2Pshutter", "DOtab"=0.0) -> (w2759:T21)
                                n386 = Array Size(array=w2760) -> (size(s)=w2758:i32)
                                n387 = Initialize Array(w2759, w2758) -> (w2757:T20)
                                n388 = call "waveformparamsv2.vi"("command"="add DO", "add DO"=w2757) -> ()  [unwired: 3 in, 3 out]
                                }
                                frame 2 {
                                # "remove False; add True"
                                n389 = call "waveformparamsv2.vi"("command"="get") -> ("Params out"=w2783:T17)  [unwired: 4 in, 2 out]
                                n390 = in-place {
                                in-place-border: w2781 -> [w2787]
                                in-place-border: [w2786] -> w2780
                                n391 = in-place-cluster #7(w2783) -> ("DO parameters"=w2789:T20)
                                n392 = for {
                                tunnel: w2787 -> [w2793] mode=indexing
                                tunnel: [w2790] -> w2786 mode=indexing
                                shift-right: [w2794] -> w2788
                                shift-left: w2789 -> [w2795]
                                n393 = Delete From Array(array=w2795, length=1, index=w2793) -> (deleted portion=w2792:T20, array with subset deleted=w2794:T20)
                                n394 = Index Array(array=w2792, index=0) -> (element=w2790:T21)
                                }
                                n395 = in-place-cluster #7("DO parameters"=w2788) -> (w2782:T17)
                                }
                                n396 = call "waveformparamsv2.vi"("command"="set", "Params in"=w2782) -> ()  [unwired: 3 in, 3 out]
                                }
                                frame 3, Default {
                                # "Remove True; Add True"
                                }
                                frame 0 {
                                # "remove False ; add False"
                                n397 = call "2pparameters.vi"("command"="get") -> ("params out"=w2801:T12)  [unwired: 1 in]
                                n398 = Unbundle By Name(w2801) -> ("autoshutter"=w2800:bool, "wavdet"=w2798:bool)
                                n399 = case shown="True" w2800 {
                                tunnel: w2799 -> [_ w2805]
                                tunnel: w2798 -> [_ w2804]
                                tunnel: [_ w2803] -> w2797
                                frame False {
                                }
                                frame True {
                                n400 = case shown="False" w2804 {
                                tunnel: w2805 -> [w2807 _]
                                tunnel: [w2806 _] -> w2803
                                frame False {
                                n401 = stacked-sequence {
                                tunnel: w2807 -> [w2809 w2816]
                                tunnel: [w2808 _] -> w2806
                                frame #0 {
                                n402 = call "waveformparamsv2.vi"("command"="get") -> ("Params out"=w2811:T17)  [unwired: 4 in, 2 out]
                                n403 = Unbundle By Name(w2811) -> ("DO parameters"=w2810:T20)
                                n404 = for {
                                tunnel: w2810 -> [w2815]
                                tunnel: w2809 -> [w2814] mode=indexing
                                tunnel: [w2813] -> w2808 mode=indexing
                                n405 = Index Array(array=w2815, index=w2814) -> (element=w2813:T21)
                                }
                                }
                                frame #1 {
                                n406 = for {
                                tunnel: w2816 -> [w2827] mode=indexing
                                w2826 = 0.0 ("padding value")
                                n407 = call "2pparameters.vi"("command"="get") -> ("params out"=w2824:T12)  [unwired: 1 in]
                                n408 = Unbundle By Name(w2824) -> ("srate"=w2821:sgl, "sAOxy"=w2823:i32)
                                n409 = To Double Precision Float(number=w2821) -> (double precision float=w2819:dbl)
                                n410 = To Double Precision Float(number=w2821) -> (double precision float=w2820:dbl)
                                n411 = To Double Precision Float(number=w2823) -> (double precision float=w2822:dbl)
                                n412 = Divide(x=w2820, y=w2822) -> (x/y=w2818:dbl)
                                n413 = call "replace DO wf param.vi"("Digital Freq (Hz)"=w2818, "Digital DC (%)"=100.0, "Digital phase"=w2826, "Sampling frequency (Hz)"=w2819, "Digital time offset (s)"=w2826, "index of DO wave"=w2827, "padding value"=w2826, "matlab wave file"=path "2Pshutter" ("matlab wave number")) -> ()  [unwired: 3 in]
                                }
                                }
                                }
                                }
                                frame True {
                                }
                                }
                                }
                                }
                                }
                                }
                              }
                              frame #7 {
                                # "... and add the actual 2p shutter waveform"
                                n414 = Build Array(w2832, w2831) -> (w2834:bool[])
                                n415 = Boolean Array To Number(Boolean array=w2834) -> (number=w2833:u32)
                                n416 = case shown="2" w2833 {
                                tunnel: w2830 -> [w2836 w2881 _ w2892]
                                tunnel: [_ w2882 _ w2890] -> w2829
                                frame 1 {
                                n417 = call "2pparameters.vi"("command"="get") -> ("params out"=w2843:T12)  [unwired: 1 in]
                                n418 = Unbundle By Name(w2843) -> ("wavdet"=w2844:bool, "sAOxy"=w2846:i32, "refwfsize"=w2847:dbl, "srate Img"=w2845:sgl)
                                n419 = call "waveformsDObuffer.vi"("command"="get") -> ("DO wf out"=w2839:digitalwaveform[])  [unwired: 1 in]
                                n420 = case shown="False" w2844 {
                                tunnel: [w2855 w2865] -> w2841
                                tunnel: w2845 -> [w2860 w2876]
                                tunnel: w2846 -> [w2854 w2869]
                                tunnel: w2847 -> [_ w2873]
                                frame False {
                                w2858 = u16 0 items=["unsigned binary", "offset binary", "2's complement"] ("data format (offset binary)")
                                n421 = Initialize Array(sgl 1.0, w2854) -> (w2851:sgl[])
                                n422 = Reciprocal(x=w2860) -> (1/x=w2861:sgl)
                                n423 = Bundle By Name("Y"=w2851, "dt"=w2861) -> (w2856:waveform(sgl))  [unwired: 1 in]
                                n424 = call-poly <vilib>:"Analog to Digital.vi"("data format (offset binary)"=w2858, "compress digital (T)"=TRUE, "full-scale range (pk-pk)"=1.0, "resolution (16 bit)"=1, "analog waveform"=w2856) -> ("digital waveform"=w2855:digitalwaveform)  [unwired: 3 in, 3 out]
                                }
                                frame True {
                                w2868 = u16 0 items=["unsigned binary", "offset binary", "2's complement"] ("data format (offset binary)")
                                n425 = To Double Precision Float(number=w2869) -> (double precision float=w2874:dbl)
                                n426 = Initialize Array(sgl 1.0, w2869) -> (w2862:sgl[])
                                n427 = Divide(x=w2873, y=w2874) -> (x/y=w2871:dbl)
                                n428 = Round Toward +Infinity(x=w2871) -> (ceil(x): smallest int >= x=w2872:dbl)
                                n429 = for {
                                N: w2872 -> [_]
                                tunnel: w2862 -> [w2878]
                                tunnel: [w2878] -> w2875 mode=concatenating
                                }
                                n430 = Reciprocal(x=w2876) -> (1/x=w2877:sgl)
                                n431 = Bundle By Name("Y"=w2875, "dt"=w2877) -> (w2866:waveform(sgl))  [unwired: 1 in]
                                n432 = call-poly <vilib>:"Analog to Digital.vi"("data format (offset binary)"=w2868, "compress digital (T)"=TRUE, "full-scale range (pk-pk)"=1.0, "resolution (16 bit)"=1, "analog waveform"=w2866) -> ("digital waveform"=w2865:digitalwaveform)  [unwired: 3 in, 3 out]
                                }
                                }
                                n433 = Array Size(array=w2836) -> (size(s)=w2835:i32)
                                n434 = for {
                                N: w2835 -> [_]
                                tunnel: w2841 -> [w2850]
                                shift-right: [w2848] -> w2837
                                shift-left: w2839 -> [w2849]
                                n435 = Build Array (concatenate)(w2849, w2850) -> (w2848:digitalwaveform[])
                                }
                                n436 = call "waveformsDObuffer.vi"("DO wf in"=w2837, "command"="set") -> ()  [unwired: 1 out]
                                }
                                frame 2 {
                                n437 = Sort 1D Array(array=w2881) -> (sorted array=w2880:i32[])
                                n438 = Reverse 1D Array(array=w2880) -> (reversed array=w2879:i32[])
                                n439 = for {
                                tunnel: w2879 -> [w2885] mode=indexing
                                tunnel: [w2884] -> w2882
                                n440 = call "waveformsDObuffer.vi"("command"="get") -> ("DO wf out"=w2887:digitalwaveform[])  [unwired: 1 in]
                                n441 = Delete From Array(array=w2887, length=1, index=w2885) -> (deleted portion=w2884:digitalwaveform[], array with subset deleted=w2883:digitalwaveform[])
                                n442 = call "waveformsDObuffer.vi"("DO wf in"=w2883, "command"="set") -> ()  [unwired: 1 out]
                                }
                                }
                                frame 3, Default {
                                }
                                frame 0 {
                                n443 = call "2pparameters.vi"("command"="get") -> ("params out"=w2894:T12)  [unwired: 1 in]
                                n444 = Unbundle By Name(w2894) -> ("autoshutter"=w2893:bool, "wavdet"=w2891:bool)
                                n445 = case shown="True" w2893 {
                                tunnel: w2892 -> [_ w2898]
                                tunnel: w2891 -> [_ w2897]
                                tunnel: [_ w2896] -> w2890
                                frame False {
                                }
                                frame True {
                                n446 = case shown="False" w2897 {
                                tunnel: w2898 -> [w2901 _]
                                tunnel: [w2900 _] -> w2896
                                frame False {
                                w2908 = u16 0 items=["unsigned binary", "offset binary", "2's complement"] ("data format (offset binary)")
                                n447 = call "2pparameters.vi"("command"="get") -> ("params out"=w2915:T12)  [unwired: 1 in]
                                n448 = call "waveformsDObuffer.vi"("command"="get") -> ("DO wf out"=w2902:digitalwaveform[])  [unwired: 1 in]
                                n449 = Unbundle By Name(w2915) -> ("sAOxy"=w2917:i32, "srate Img"=w2916:sgl)
                                n450 = Initialize Array(sgl 1.0, w2917) -> (w2903:sgl[])
                                n451 = Reciprocal(x=w2916) -> (1/x=w2910:sgl)
                                n452 = Bundle By Name("Y"=w2903, "dt"=w2910) -> (w2906:waveform(sgl))  [unwired: 1 in]
                                n453 = call-poly <vilib>:"Analog to Digital.vi"("data format (offset binary)"=w2908, "compress digital (T)"=TRUE, "full-scale range (pk-pk)"=1.0, "resolution (16 bit)"=1, "analog waveform"=w2906) -> ("digital waveform"=w2913:digitalwaveform)  [unwired: 3 in, 3 out]
                                n454 = for {
                                tunnel: w2913 -> [w2922]
                                tunnel: w2901 -> [w2919] mode=indexing
                                tunnel: [w2918] -> w2900 mode=indexing
                                shift-right: [w2920] -> w2899
                                shift-left: w2902 -> [w2921]
                                n455 = Index Array(array=w2921, index=w2919) -> (element=w2918:digitalwaveform)
                                n456 = Replace Array Subset(array=w2921, new element=w2922, index=w2919) -> (w2920:digitalwaveform[])
                                }
                                n457 = call "waveformsDObuffer.vi"("DO wf in"=w2899, "command"="set") -> ()  [unwired: 1 out]
                                }
                                frame True {
                                }
                                }
                                }
                                }
                                }
                                }
                              }
                              frame #8 {
                                # "Calculate lifetime timestamp waveform"
                                n458 = Build Array(w2926, w2925) -> (w2928:bool[])
                                n459 = Boolean Array To Number(Boolean array=w2928) -> (number=w2927:u32)
                                n460 = case shown="0" w2927 {
                                tunnel: w2924 -> [_ w2954 _ w2966]
                                tunnel: [_ w2953 _ w2964] -> w2923
                                frame 1 {
                                w2941 = 0.0 ("DOtab")
                                n461 = call "2pparameters.vi"("command"="get") -> ("params out"=w2939:T12)  [unwired: 1 in]
                                n462 = call "waveformparamsv2.vi"("command"="get") -> ("Params out"=w2949:T17)  [unwired: 4 in, 2 out]
                                n463 = Unbundle By Name(w2949) -> ("DO parameters"=w2947:T20)
                                n464 = Unbundle By Name(w2939) -> ("srate"=w2936:sgl, "sAOxy"=w2938:i32)
                                n465 = To Double Precision Float(number=w2936) -> (double precision float=w2934:dbl)
                                n466 = To Double Precision Float(number=w2936) -> (double precision float=w2935:dbl)
                                n467 = To Double Precision Float(number=w2938) -> (double precision float=w2930:dbl)
                                n468 = Divide(x=w2935, y=w2930) -> (x/y=w2937:dbl)
                                n469 = Index Array(array=w2947, index=0) -> (element=w2946:T21)
                                n470 = Divide(x=1.0 ("Digital DC (%)"), y=w2930) -> (x/y=w2932:dbl)
                                n471 = Multiply(x=100.0, y=w2932) -> (x*y=w2929:dbl)
                                n472 = Bundle By Name(cluster=w2946, "Digital DC (%)"=w2929, "Digital phase"=w2941, "Digital Freq (Hz)"=w2937, "Sampling frequency (Hz)"=w2934, "Digital time offset (s)"=w2941, "padding value"=0.0, "matlab wave file"=path "LT", "DOtab"=0.0) -> (w2944:T21)
                                n473 = Build Array(w2944) -> (w2943:T20)
                                n474 = call "waveformparamsv2.vi"("command"="add DO", "add DO"=w2943) -> ()  [unwired: 3 in, 3 out]
                                }
                                frame 2 {
                                n475 = call "waveformparamsv2.vi"("command"="get") -> ("Params out"=w2956:T17)  [unwired: 4 in, 2 out]
                                n476 = in-place {
                                in-place-border: w2954 -> [w2960]
                                in-place-border: [w2959] -> w2953
                                n477 = in-place-cluster #8(w2956) -> ("DO parameters"=w2962:T20)
                                n478 = Delete From Array(array=w2962, length=1, index=w2960) -> (deleted portion=w2959:T20, array with subset deleted=w2961:T20)
                                n479 = in-place-cluster #8("DO parameters"=w2961) -> (w2955:T17)
                                }
                                n480 = call "waveformparamsv2.vi"("command"="set", "Params in"=w2955) -> ()  [unwired: 3 in, 3 out]
                                }
                                frame 3, Default {
                                }
                                frame 0 {
                                n481 = local read "Measurement"() -> (w2968:T4)
                                n482 = To Unsigned Long Integer(number=w2968) -> (unsigned 32bit integer=w2967:u32)
                                n483 = case shown="5..7" w2967 {
                                tunnel: w2966 -> [_ w2970]
                                tunnel: [_ w2969] -> w2965
